vi "generator2.vi"() -> ()   [LabVIEW 2025]
uses:
  <vilib>/measure/NI_MABase.lvlib
panel:
  out "Waveform Graph":waveform(dbl)(graph)
  out "Fs":dbl format="%#_13g"
  out "Nyquist Eqn":string
  out "cycle of signals":i32
  in  "stop":bool
  in  "amplitude  noise 2":dbl(knob)=1.0 min=0.001 max=1.0 step=0.1 scale=0.001..1.0
  in  "frequency 2":dbl(knob)=100.0 min=100.0 max=10000.0 step=10.0 scale=100.0..10000.0
  in  "amplitude 2":dbl(knob)=1.0 min=0.1 max=10.0 step=0.1 scale=0.1..10.0
  in  "phase 2":dbl(slide) min=0.0 max=360.0 step=5.0 scale=0.0..360.0
  in  "signal type 2":T1(ring)
  in  "sampling info 2":cluster{"Fs":dbl, "#s":dbl}={"Fs"=1000.0, "#s"=1000.0} {"Fs" format="%.2p"}
  in  "square wave duty cycle (%) 2":dbl=50.0 format="%0.2f"
  in  "offset 2":dbl(slide)=0.005 min=0.005 max=5.0 step=0.1 scale=0.005..5.0
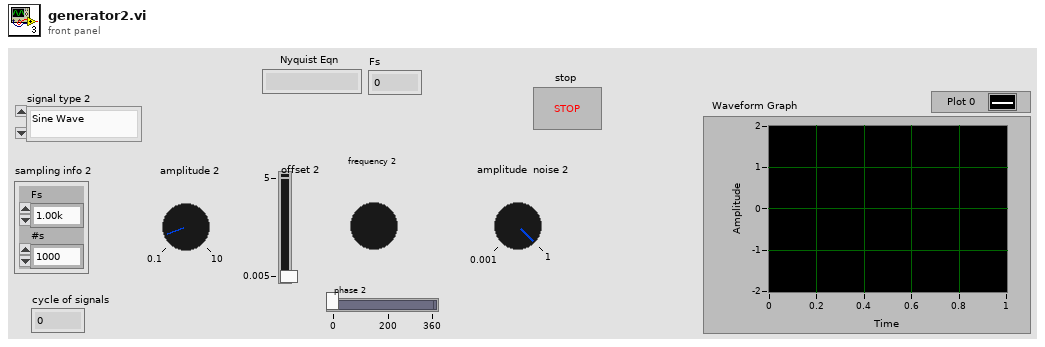
[diagram p1: front panel]
types:
  T1 = enum16{"Sine Wave", "Triangle Wave", "Square Wave", "Sawtooth Wave"}
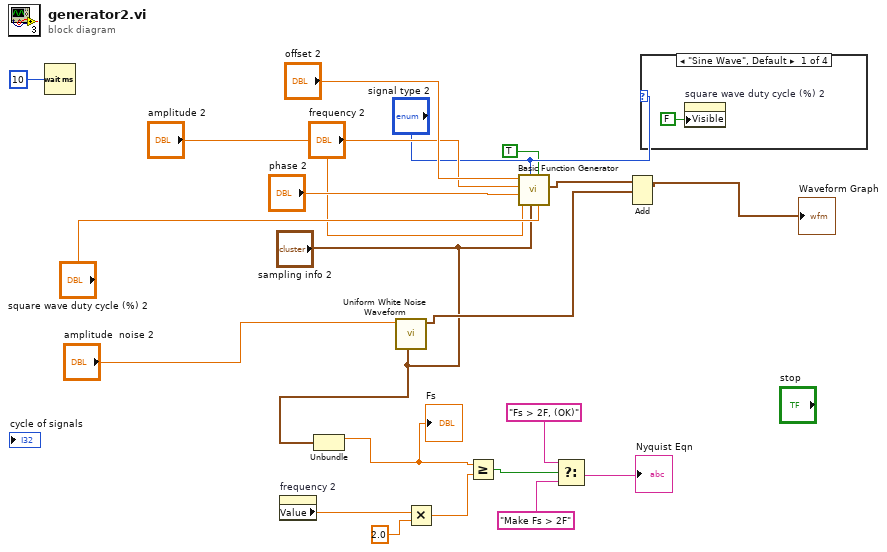
[diagram p0: block diagram]
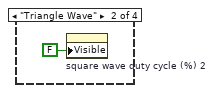
[diagram p2: hidden frame]
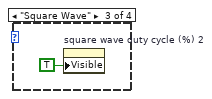
[diagram p3: hidden frame]
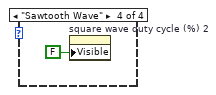
[diagram p4: hidden frame]
diagram:
  n1 = Wait (ms)(milliseconds to wait=10) -> ()  [unwired: 1 out]
  n2 = property on="frequency 2" class="Knob (strict)"() -> ("Value"=w5:dbl)  [unwired: 2 in, 2 out]
  n3 = Unbundle("sampling info 2") -> ("Fs"=w3:dbl)  [unwired: 1 out]
  "Fs" <- w3
  n4 = call <vilib>:"Uniform White Noise Waveform.vi"("sampling info"="sampling info 2", "amplitude"="amplitude  noise 2") -> ("signal out"=w13:waveform(dbl))  [unwired: 8 in, 1 out]
  n5 = Multiply(x=w5, y=2.0) -> (x*y=w7:dbl)
  n6 = Greater Or Equal?(x=w3, y=w7) -> (x >= y?=w9:bool)
  n7 = call <vilib>:"Basic Function Generator.vi"("offset"="offset 2", "square wave duty cycle (%)"="square wave duty cycle (%) 2", "reset signal"=TRUE, "sampling info"="sampling info 2", "signal type"="signal type 2", "phase"="phase 2", "amplitude"="amplitude 2", "frequency"="frequency 2") -> ("signal out"=w14:waveform(dbl))  [unwired: 1 in, 2 out]
  n8 = Select(t="Fs > 2F, (OK)", s=w9, f="Make Fs > 2F") -> (s? t:f=→"Nyquist Eqn":string)
  n9 = Add(1:w13, 2:w14) -> (0:→"Waveform Graph":waveform(dbl))  [unwired: 1 in, 1 out]
  n10 = case shown="\"Sine Wave\", Default" "signal type 2" {
    frame "Sine Wave", Default {
      n11 = property on="square wave duty cycle (%) 2" class="DigNum (strict)"("Visible"=FALSE) -> ()  [unwired: 2 in, 2 out]
    }
    frame "Triangle Wave" {
      n12 = property on="square wave duty cycle (%) 2" class="DigNum (strict)"("Visible"=FALSE) -> ()  [unwired: 2 in, 2 out]
    }
    frame "Square Wave" {
      n13 = property on="square wave duty cycle (%) 2" class="DigNum (strict)"("Visible"=TRUE) -> ()  [unwired: 2 in, 2 out]
    }
    frame "Sawtooth Wave" {
      n14 = property on="square wave duty cycle (%) 2" class="DigNum (strict)"("Visible"=FALSE) -> ()  [unwired: 2 in, 2 out]
    }
  }
